vi "SpielFeldInitial(SubVI).vi"(0 "SpalteUndZeile":u8) -> (1 "TictactoeFelder":bool[][](array[boolean]), 2 "Grafikring":i8[][](array[numeric]))   [LabVIEW 2017]
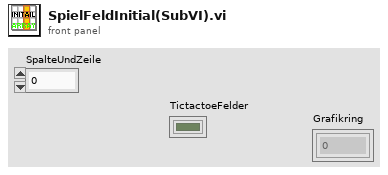
[diagram p1: front panel]
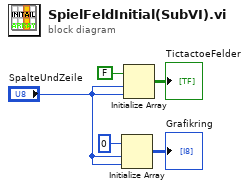
[diagram p0: block diagram]
diagram:
  n1 = Initialize Array(0, "SpalteUndZeile", "SpalteUndZeile") -> (→"Grafikring":i32[][])
  n2 = Initialize Array(FALSE, "SpalteUndZeile", "SpalteUndZeile") -> (→"TictactoeFelder":bool[][])
